vi "workspace.get_details.vi"(8 "error in":errorcluster, 10 "Workspace RID":string, 11 "Nominal Client in":refnum<class "Nominal Client.lvclass">) -> (0 "error out":errorcluster, 1 "Workspace Details":T1, 2 "Workspace RID":string, 3 "Nominal Client out":refnum<class "Nominal Client.lvclass">)   [LabVIEW 2020, in "Nominal Client.lvclass"]
doc: "Gets the workspace with the specified WorkspaceRid."
uses:
  Nominal Client.lvclass
  ce527530-f409-488f-b07f-3b5ecba8805e.vi
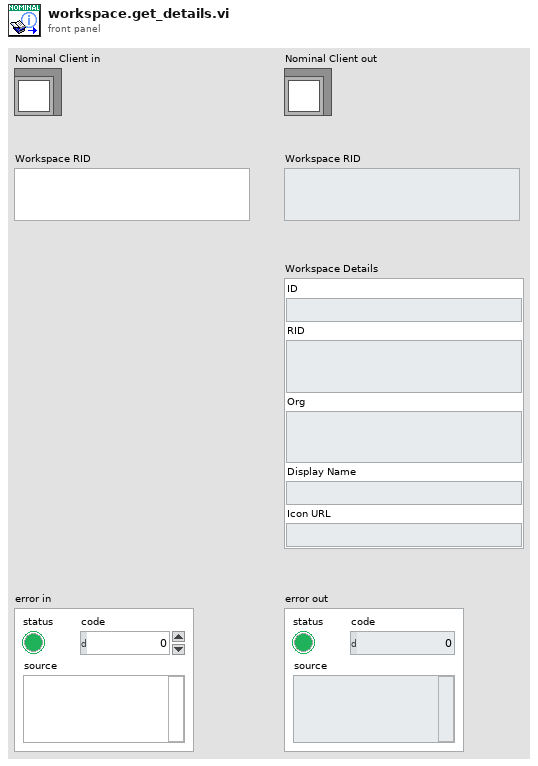
[diagram p1: front panel]
types:
  T1 = cluster{"ID":string, "RID":string, "Org":string, "Display Name":string, "Icon URL":string}
  T2 = cluster{"id":string, "rid":string, "org":string, "displayName":string, "iconUrl":string}
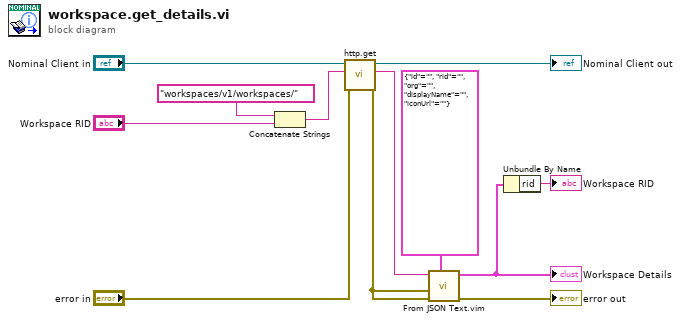
[diagram p0: block diagram]
diagram:
  n1 = Concatenate Strings("workspaces/v1/workspaces/" ("Path"), "Workspace RID") -> (w4:string)
  n2 = call "http.get.vi"("error in"="error in", "Path"=w4, "Nominal Client in"="Nominal Client in") -> ("error out"=w7:errorcluster, "Response"=w8:string, "Nominal Client out"=→"Nominal Client out":refnum<class "Nominal Client.lvclass">)  [unwired: 5 in, 1 out]
  "error out" <- w7
  n3 = call "From JSON Text.vim"("Data Type and Default Value"=T2 {"id"="", "rid"="", "org"="", "displayName"="", "iconUrl"=""} ("Workspace"), "error in (no error)"=w7, "JSON"=w8) -> ("Data out"=w2:T2)  [unwired: 7 in, 1 out]
  "Workspace Details" <- w2
  n4 = Unbundle By Name(w2) -> ("rid"=→"Workspace RID":string)
